vi "macro_SwerveDriveKineNewX.vi"   [LabVIEW 2019, in "Trajectory_Library.lvlib"]
uses:
  Trajectory_Library.lvlib
types:
  T1 = typedef "WPILib_Math.lvlib/TRANSLATION2D.ctl" = cluster{"X":dbl, "Y":dbl}
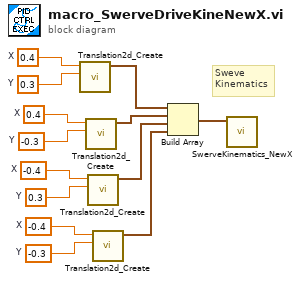
[diagram p0: block diagram]
diagram:
  w6 = -0.4  # X
  w7 = -0.3  # Y
  w8 = -0.4  # X
  w9 = 0.3  # Y
  w10 = 0.4  # X
  w11 = -0.3  # Y
  w12 = 0.4  # X
  w13 = 0.3  # Y
  # "Sweve\nKinematics"
  n1 = call "Translation2d_Create.vi"("Y"=w13, "X"=w12) -> ("TRANSLATION"=w2:T1)  [unwired: 9 in]
  n2 = call "Translation2d_Create.vi"("Y"=w11, "X"=w10) -> ("TRANSLATION"=w3:T1)  [unwired: 9 in]
  n3 = call "Translation2d_Create.vi"("Y"=w9, "X"=w8) -> ("TRANSLATION"=w4:T1)  [unwired: 9 in]
  n4 = call "Translation2d_Create.vi"("Y"=w7, "X"=w6) -> ("TRANSLATION"=w5:T1)  [unwired: 9 in]
  n5 = Build Array(w2, w3, w4, w5) -> (w1:T1[])
  n6 = call "SwerveKinematics_NewX.vi"("Wheels"=w1) -> ()  [unwired: 10 in, 1 out]
